vi "Linear Length 2 1478 1525 1828.vi"(0 "Input Image":T2, 1 "Calibration Image":T2, 5 "Ref ROI Parameters":T9={"Ref ROI After Transformation"={"Global Rectangle"=[], "Contours"=[]}, "Ref ROI Edge Options"={"Edge Polarity"=0, "Kernel Size"=3, "Width"=3, "Minimum Edge Strength"=10.0, "Interpolation Type"=enum."Zero Order", "Data Processing Method"=enum."Average"}, "Ref ROI Line Options"={"Number of Lines"=1, "Type"=enum."Best Edge Projection", "Min. Score"=0.0, "Max. Score"=1000.0, "Orientation"=0.0, "Angle Range"=5.0, "Angle Tolerance"=0.0, "Step Size"=5, "Min. SNR (db)"=0.0, "Min. Points (%)"=25.0, "Hough Iterations"=5}, "Ref ROI Search Direction"=0, "Ref ROI Overlay"=FALSE} {"Ref ROI Edge Options"."Edge Polarity" items=["All Edges", "Rising Edges", "Falling Edges"]; "Ref ROI Edge Options"."Minimum Edge Strength" format="%.2f"; "Ref ROI Edge Options"."Width" step=2; "Ref ROI Edge Options"."Kernel Size" step=2; "Ref ROI Line Options"."Min. Points (%)" min=0.0 max=100.0; "Ref ROI Line Options"."Min. SNR (db)" min=0.0; "Ref ROI Line Options"."Max. Score" min=0.0 max=1024.0; "Ref ROI Line Options"."Min. Score" min=0.0 max=1024.0 step=1.0}, 7 "ROI 1 Parameters":T6={"ROI 1 After Transformation"={"Global Rectangle"=[], "Contours"=[]}, "ROI 1 Edge Options"={"Edge Polarity"=0, "Kernel Size"=3, "Width"=3, "Minimum Edge Strength"=10.0, "Interpolation Type"=enum."Bilinear Fixed", "Data Processing Method"=enum."Average"}, "ROI 1 Scan Direction"=0, "ROI 1 Step Size"=0, "ROI 1 Process"=enum."Get First Edge", "ROI 1 Overlay"=FALSE, "ROI 1 Rake Line Overlay"=FALSE, "ROI 1 Edge/Point Overlay"=FALSE} {"ROI 1 Edge Options"."Edge Polarity" items=["All Edges", "Rising Edges", "Falling Edges"]; "ROI 1 Edge Options"."Minimum Edge Strength" format="%.2f"; "ROI 1 Edge Options"."Width" step=2; "ROI 1 Edge Options"."Kernel Size" step=2}, 9 "ROI 2 Parameters":T5={"ROI 2 After Transformation"={"Global Rectangle"=[], "Contours"=[]}, "ROI 2 Edge Options"={"Edge Polarity"=0, "Kernel Size"=3, "Width"=3, "Minimum Edge Strength"=10.0, "Interpolation Type"=enum."Bilinear Fixed", "Data Processing Method"=enum."Average"}, "ROI 2 Scan Direction"=0, "ROI 2 Step Size"=0, "ROI 2 Process"=enum."Get First Edge", "ROI 2 Overlay"=FALSE, "ROI 2 Rake Line Overlay"=FALSE, "ROI 2 Edge/Point Overlay"=FALSE} {"ROI 2 Edge Options"."Edge Polarity" items=["All Edges", "Rising Edges", "Falling Edges"]; "ROI 2 Edge Options"."Minimum Edge Strength" format="%.2f"; "ROI 2 Edge Options"."Width" step=2; "ROI 2 Edge Options"."Kernel Size" step=2}, 11 "error in (no error)":errorcluster) -> (4 "Refnum out":T2(plugin-control), 6 "output cluster":T10, 8 "Overlay Arrow Lines":T1, 15 "error out":errorcluster)   [LabVIEW 2019, in "Algorithm.lvclass"]
uses:
  FrameworkOverrides/Algorithm.lvclass
  <vilib>/vision/NI_Vision_Development_Module.lvlib
  <vilib>/vision/Measure.llb/Edge Polarity.ctl
  <vilib>/vision/Measure.llb/Edge Options.ctl
  <vilib>/vision/Measure.llb/Straight Edge Process.ctl
  <vilib>/vision/Measure.llb/Straight Edge Options.ctl
  <vilib>/vision/Image Controls.llb/IMAQ Image.ctl
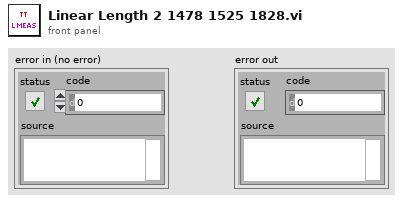
[diagram p1: front panel]
types:
  T1 = cluster{cluster{cluster{sgl, "Y":sgl}, "Point 2":cluster{"X":sgl, "Y":sgl}}, cluster{"Point 2":cluster{"X":sgl, "Y":sgl}, cluster{sgl, "Y":sgl}}}
  T2 = typedef "IMAQ Image.ctl" = refnum<image>
  T3 = typedef "Edge Options.ctl" = cluster{"Edge Polarity":T4, "Kernel Size":u32, "Width":u32, "Minimum Edge Strength":sgl, "Interpolation Type":enum32{"Zero Order", "Bilinear", "Quadratic", "Cubic", "Bilinear Fixed"}, "Data Processing Method":enum32{"Average", "Median"}}
  T4 = typedef "Edge Polarity.ctl" = u32
  T5 = cluster{"ROI 2 After Transformation":cluster{"Global Rectangle":i32[], "Contours":cluster{"ID":enum32{"External", "Internal"}, "Type":u32, "Coordinates":i32[]}[]}, "ROI 2 Edge Options":T3, "ROI 2 Scan Direction":u16, "ROI 2 Step Size":u32, "ROI 2 Process":enum16{"Get First Edge", "Get First + Last Edge", "Get All Edges", "Get Best Edge"}, "ROI 2 Overlay":bool, "ROI 2 Rake Line Overlay":bool, "ROI 2 Edge/Point Overlay":bool}
  T6 = cluster{"ROI 1 After Transformation":cluster{"Global Rectangle":i32[], "Contours":cluster{"ID":enum32{"External", "Internal"}, "Type":u32, "Coordinates":i32[]}[]}, "ROI 1 Edge Options":T3, "ROI 1 Scan Direction":u16, "ROI 1 Step Size":u32, "ROI 1 Process":enum16{"Get First Edge", "Get First + Last Edge", "Get All Edges", "Get Best Edge"}, "ROI 1 Overlay":bool, "ROI 1 Rake Line Overlay":bool, "ROI 1 Edge/Point Overlay":bool}
  T7 = typedef "Straight Edge Options.ctl" = cluster{"Number of Lines":i32, "Type":T8, "Min. Score":dbl, "Max. Score":dbl, "Orientation":dbl, "Angle Range":dbl, "Angle Tolerance":dbl, "Step Size":u32, "Min. SNR (db)":dbl, "Min. Points (%)":dbl, "Hough Iterations":i32}
  T8 = typedef "Straight Edge Process.ctl" = enum32{"First Edge Rake", "Best Edge Rake", "Hough Edge Rake", "First Edge Projection", "Best Edge Projection"}
  T9 = cluster{"Ref ROI After Transformation":cluster{"Global Rectangle":i32[], "Contours":cluster{"ID":enum32{"External", "Internal"}, "Type":u32, "Coordinates":i32[]}[]}, "Ref ROI Edge Options":T3, "Ref ROI Line Options":T7, "Ref ROI Search Direction":u32, "Ref ROI Overlay":bool}
  T10 = cluster{"L Meas":sgl, "output cluster":cluster{"Point 2":cluster{"X":sgl, "Y":sgl}, "Point 2":cluster{"X":sgl, "Y":sgl}}}
  T11 = cluster{"First Overlay Line ":cluster{"Start Point":cluster{"X":sgl, "Y":sgl}, "Start Point":cluster{"X":sgl, "Y":sgl}}, "Second Overlay Line ":cluster{"Start Point":cluster{"X":sgl, "Y":sgl}, "Start Point":cluster{"X":sgl, "Y":sgl}}}
  T12 = cluster{"Search Direction":u32, "Edge Options":T3, "Show Search Area":bool, "Show Search Lines":bool, "Show Edges Found":bool, "Show Result":bool, "Search Area Color":u32, "Search Lines Color":u32, "Edge Locations Color":u32, "Result Color":u32, "Overlay Group Name":string}
  T13 = cluster{"Global Rectangle":i32[], "Contours":cluster{"ID":enum32{"External", "Internal"}, "Type":u32, "Coordinates":i32[]}[]}
  T14 = enum16{"Get First Edge", "Get First + Last Edge", "Get All Edges", "Get Best Edge"}
  T15 = cluster{"Point1 (Pixels)":cluster{"X":sgl, "Y":sgl}, "Point2 (Pixels)":cluster{"X":sgl, "Y":sgl}, "Point1 (Real-World)":cluster{"X":sgl, "Y":sgl}, "Point2 (Real-World)":cluster{"X":sgl, "Y":sgl}, "Angle (Pixel)":dbl, "Angle (Real-World)":dbl, "Score":dbl, "Straightness":dbl, "Average SNR (db)":dbl, "Calibration Valid":bool}[]
  T16 = typedef "Edge New.ctl" = cluster{"Location (Pixel)":cluster{"X":sgl, "Y":sgl}, "Location (Real-World)":cluster{"X":sgl, "Y":sgl}, "Distance (Pixel)":dbl, "Distance (Real-World)":dbl, "Strength":dbl, "Noise":dbl, "Rising?":bool}
  T17 = typedef "Search Line.ctl" = cluster{"Start Point":cluster{"X":sgl, "Y":sgl}, "End Point":cluster{"X":sgl, "Y":sgl}, "Edge Info":T16[], "Edge Map":dbl[], "Calibration Valid":bool}
  T18 = cluster{"Point1 (Pixels)":cluster{"X":sgl, "Y":sgl}, "Point2 (Pixels)":cluster{"X":sgl, "Y":sgl}, "Point1 (Real-World)":cluster{"X":sgl, "Y":sgl}, "Point2 (Real-World)":cluster{"X":sgl, "Y":sgl}, "Angle (Pixel)":dbl, "Angle (Real-World)":dbl, "Score":dbl, "Straightness":dbl, "Average SNR (db)":dbl, "Calibration Valid":bool}
  T19 = cluster{"Point1 (Pixels)":cluster{"X":sgl, "Y":sgl}, "Point2 (Pixels)":cluster{"X":sgl, "Y":sgl}}
  T20 = cluster{"Point 1":cluster{"X":sgl, "Y":sgl}, "Point 2":cluster{"X":sgl, "Y":sgl}}
  T21 = cluster{"Point 2":cluster{"X":sgl, "Y":sgl}, "Point 2":cluster{"X":sgl, "Y":sgl}}
  T22 = cluster{cluster{sgl, "Y":sgl}, "Point 2":cluster{"X":sgl, "Y":sgl}}
  T23 = cluster{"Point 2":cluster{"X":sgl, "Y":sgl}, cluster{sgl, "Y":sgl}}
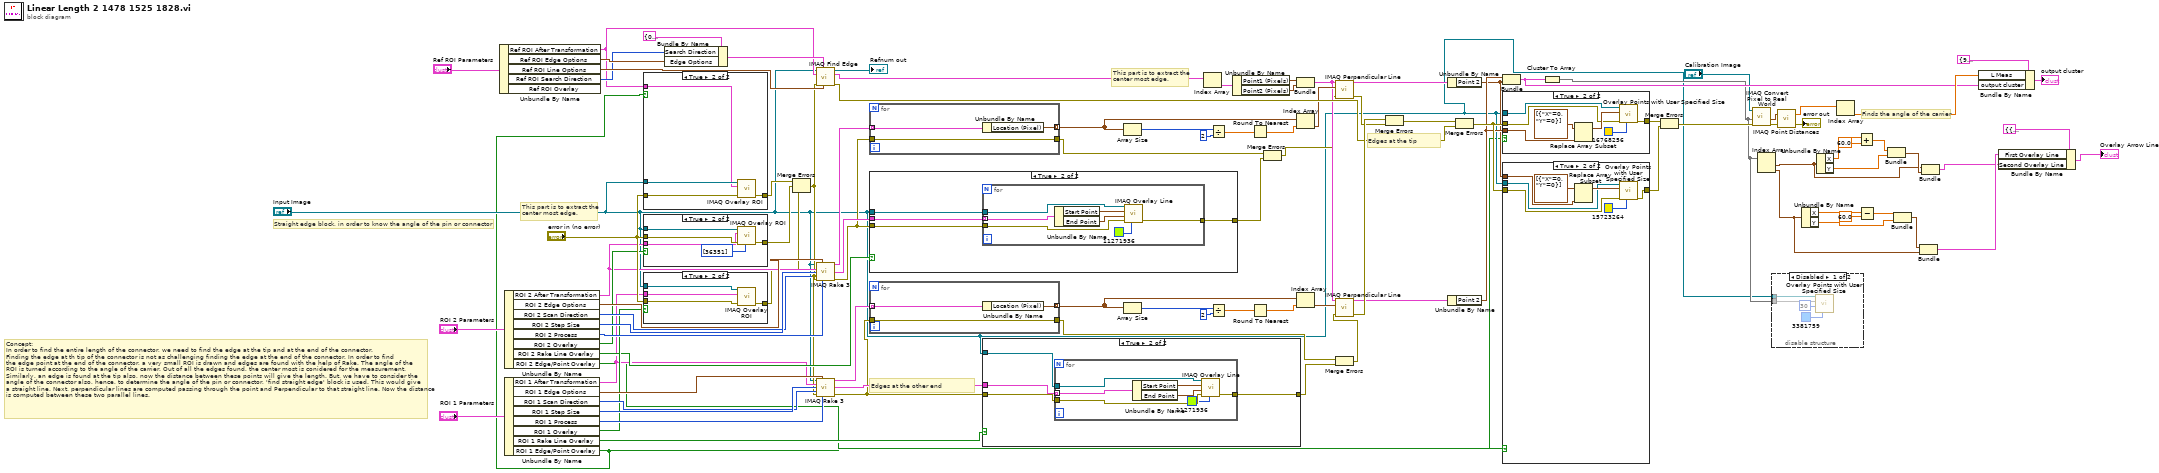
[diagram p0: block diagram]
diagram:
  # "Straight edge block, in order to know the angle of the pin or connector"
  # "This part is to extract the\ncenter most edge."
  # "This part is to extract the\ncenter most edge."
  # "Concept:\nIn order to find the entire length of the connector, we need to find the edge at the tip and at the end of the connector.\nFinding the edge at th tip of the connector is not as challenging finding the edge at the end of the connector. In order to find\nthe edge point at the end of the connector, a very small ROI is drawn and edges are found with the help of Rake. The angle of the \nROI is turned according to the angle of the carrier. Out of all the edges found, the center most is conidered for the measurement.\nSimilarly, an edge is found at the tip also, now the distance between these points will give the length. But, we have to consider the \nangle of the connector also, hence, to determine the angle of the pin or connector, 'find straight edge' block is used. This would give\na straight line. Next, perpendicular lines are computed passing through the point and Perpendicular to that straight line. Now the distance\nis computed between these two parallel lines."
  # "Finds the angle of the carrier"
  # "Edges at the other end"
  # "Edges at the tip"
  n1 = Unbundle By Name("Ref ROI Parameters") -> ("Ref ROI After Transformation"=w36:T13, "Ref ROI Edge Options"=w65:T3, "Ref ROI Line Options"=w66:T7, "Ref ROI Search Direction"=w64:u32)  [unwired: 1 out]
  n2 = Unbundle By Name("ROI 2 Parameters") -> ("ROI 2 After Transformation"=w47:T13, "ROI 2 Edge Options"=w63:T3, "ROI 2 Scan Direction"=w60:u16, "ROI 2 Step Size"=w61:u32, "ROI 2 Process"=w62:T14, "ROI 2 Overlay"=w48:bool, "ROI 2 Rake Line Overlay"=w44:bool, "ROI 2 Edge/Point Overlay"=w35:bool)
  n3 = Unbundle By Name("ROI 1 Parameters") -> ("ROI 1 After Transformation"=w37:T13, "ROI 1 Edge Options"=w59:T3, "ROI 1 Scan Direction"=w56:u16, "ROI 1 Step Size"=w57:u32, "ROI 1 Process"=w58:T14, "ROI 1 Overlay"=w50:bool, "ROI 1 Rake Line Overlay"=w43:bool, "ROI 1 Edge/Point Overlay"=w1:bool)
  n4 = case shown="True" w1 {
    tunnel: "error in (no error)" -> [w100 w104]
    tunnel: [w100 w103] -> w32
    tunnel: "Input Image" -> [_ w102]
    tunnel: w36 -> [_ w101]
    frame False {
    }
    frame True {
      n5 = call "IMAQ Overlay ROI"("error in (no error)"=w104, "ROI Descriptor"=w101, "Image"=w102) -> ("error out"=w103:errorcluster)  [unwired: 7 in, 1 out]
    }
  }
  n6 = case shown="True" w48 {
    tunnel: "error in (no error)" -> [w105 w110]
    tunnel: [w105 w109] -> w31
    tunnel: "Input Image" -> [_ w108]
    tunnel: w47 -> [_ w107]
    frame False {
    }
    frame True {
      n7 = call "IMAQ Overlay ROI"("Colors (Green)"=u32[] [36351], "error in (no error)"=w110, "ROI Descriptor"=w107, "Image"=w108) -> ("error out"=w109:errorcluster)  [unwired: 6 in, 1 out]
    }
  }
  n8 = case shown="True" w50 {
    tunnel: "error in (no error)" -> [w111 w115]
    tunnel: [w111 w114] -> w30
    tunnel: "Input Image" -> [_ w113]
    tunnel: w37 -> [_ w112]
    frame False {
    }
    frame True {
      n9 = call "IMAQ Overlay ROI"("error in (no error)"=w115, "ROI Descriptor"=w112, "Image"=w113) -> ("error out"=w114:errorcluster)  [unwired: 7 in, 1 out]
    }
  }
  n10 = Bundle By Name(cluster=T12 {"Search Direction"=0, "Edge Options"={"Edge Polarity"=0, "Kernel Size"=3, "Width"=3, "Minimum Edge Strength"=10.0, "Interpolation Type"=enum."Bilinear Fixed", "Data Processing Method"=enum."Average"}, "Show Search Area"=FALSE, "Show Search Lines"=FALSE, "Show Edges Found"=FALSE, "Show Result"=TRUE, "Search Area Color"=65280, "Search Lines Color"=255, "Edge Locations Color"=16776960, "Result Color"=65337, "Overlay Group Name"=""} ("Options"), "Search Direction"=w64, "Edge Options"=w65) -> (w70:T12)
  n11 = Merge Errors(w32, w31, w30) -> (w29:errorcluster)
  n12 = call "IMAQ Find Edge"("Line Fit Options"=w66, "Options"=w70, "error in (no error)"=w29, "ROI Descriptor"=w36, "Image"="Input Image") -> ("error out"=w95:errorcluster, "Straight Edges"=w90:T15, "Image Out"=→"Refnum out":T2)  [unwired: 3 in, 1 out]
  n13 = call "IMAQ Rake 3"("Image"="Input Image", "Edge Options"=w63, "ROI Descriptor"=w47, "Step Size"=w61, "Scan Direction"=w60, "error in (no error)"=w29, "Process"=w62) -> ("First Edges"=w81:T16[], "Search Lines"=w45:T17[], "error out"=w28:errorcluster)  [unwired: 5 in, 1 out]
  n14 = call "IMAQ Rake 3"("Image"="Input Image", "Edge Options"=w59, "ROI Descriptor"=w37, "Step Size"=w57, "Scan Direction"=w56, "error in (no error)"=w29, "Process"=w58) -> ("First Edges"=w20:T16[], "Search Lines"=w46:T17[], "error out"=w22:errorcluster)  [unwired: 5 in, 1 out]
  n15 = for {
    tunnel: w81 -> [w118] mode=indexing
    tunnel: [w117] -> w73 mode=indexing
    tunnel: w28 -> [w116]
    tunnel: [w116] -> w27
    n16 = Unbundle By Name(w118) -> ("Location (Pixel)"=w117:cluster{"X":sgl, "Y":sgl})
  }
  n17 = case shown="True" w44 {
    tunnel: [w119 w123] -> w26
    tunnel: w28 -> [w119 w122]
    tunnel: w45 -> [_ w121]
    tunnel: "Input Image" -> [_ w120]
    frame False {
    }
    frame True {
      n18 = for {
        tunnel: [w130] -> w123
        tunnel: w122 -> [w129]
        tunnel: w121 -> [w128] mode=indexing
        tunnel: w120 -> [w125]
        n19 = Unbundle By Name(w128) -> ("Start Point"=w127:cluster{"X":sgl, "Y":sgl}, "End Point"=w126:cluster{"X":sgl, "Y":sgl})
        n20 = call "IMAQ Overlay Line"("Color"=u32 11271936, "error in (no error)"=w129, "End Point"=w126, "Start Point"=w127, "Image"=w125) -> ("error out"=w130:errorcluster)  [unwired: 5 in, 1 out]
      }
    }
  }
  n21 = for {
    tunnel: w20 -> [w133] mode=indexing
    tunnel: [w132] -> w52 mode=indexing
    tunnel: w22 -> [w131]
    tunnel: [w131] -> w21
    n22 = Unbundle By Name(w133) -> ("Location (Pixel)"=w132:cluster{"X":sgl, "Y":sgl})
  }
  n23 = case shown="True" w43 {
    tunnel: [w134 w138] -> w24
    tunnel: w22 -> [w134 w137]
    tunnel: w46 -> [_ w136]
    tunnel: "Input Image" -> [_ w135]
    frame False {
    }
    frame True {
      n24 = for {
        tunnel: [w145] -> w138
        tunnel: w137 -> [w144]
        tunnel: w136 -> [w143] mode=indexing
        tunnel: w135 -> [w140]
        n25 = Unbundle By Name(w143) -> ("Start Point"=w142:cluster{"X":sgl, "Y":sgl}, "End Point"=w141:cluster{"X":sgl, "Y":sgl})
        n26 = call "IMAQ Overlay Line"("Color"=u32 11271936, "error in (no error)"=w144, "End Point"=w141, "Start Point"=w142, "Image"=w140) -> ("error out"=w145:errorcluster)  [unwired: 5 in, 1 out]
      }
    }
  }
  n27 = Array Size(array=w73) -> (size(s)=w89:i32)
  n28 = Array Size(array=w52) -> (size(s)=w82:i32)
  n29 = Index Array(array=w90) -> (element=w91:T18)  [unwired: 1 in]
  n30 = Divide(x=w89, y=2 ("index (row)")) -> (x/y=w87:dbl)
  n31 = Divide(x=w82, y=2 ("index (row)")) -> (x/y=w84:dbl)
  n32 = Unbundle By Name(w91) -> ("Point1 (Pixels)"=w75:cluster{"X":sgl, "Y":sgl}, "Point2 (Pixels)"=w74:cluster{"X":sgl, "Y":sgl})
  n33 = Round To Nearest(number=w87) -> (nearest integer value=w86:dbl)
  n34 = Round To Nearest(number=w84) -> (nearest integer value=w85:dbl)
  n35 = Merge Errors(w27, w26) -> (w25:errorcluster)
  n36 = Bundle("Point1 (Pixels)"=w75, "Point2 (Pixels)"=w74) -> (w92:T19)  [unwired: 1 in]
  n37 = Index Array(array=w73, index=w86) -> (element=w94:cluster{"X":sgl, "Y":sgl})
  n38 = Index Array(array=w52, index=w85) -> (element=w93:cluster{"X":sgl, "Y":sgl})
  n39 = call "IMAQ Perpendicular Line"("error in (no error)"=w25, "Point"=w94, "Line"=w92) -> ("error out"=w96:errorcluster, "Perpendicular Line"=w53:T20)  [unwired: 6 in, 1 out]
  n40 = Merge Errors(w21, w24) -> (w23:errorcluster)
  n41 = call "IMAQ Perpendicular Line"("error in (no error)"=w23, "Point"=w93, "Line"=w92) -> ("error out"=w97:errorcluster, "Perpendicular Line"=w54:T20)  [unwired: 6 in, 1 out]
  n42 = Merge Errors(w97, w96) -> (w98:errorcluster)
  n43 = Unbundle By Name(w53) -> ("Point 2"=w38:cluster{"X":sgl, "Y":sgl})
  n44 = Unbundle By Name(w54) -> ("Point 2"=w39:cluster{"X":sgl, "Y":sgl})
  n45 = Merge Errors(w98, w95) -> (w40:errorcluster)
  n46 = Bundle("Point 2"=w39, "Point 2"=w38) -> (w76:T21)  [unwired: 1 in]
  n47 = case shown="True" w1 {
    tunnel: [w146 w150] -> w42
    tunnel: w40 -> [w146 w151]
    tunnel: w39 -> [_ w149]
    tunnel: "Input Image" -> [_ w148]
    frame False {
    }
    frame True {
      n48 = Replace Array Subset(array=cluster{"X":i32, "Y":i32}[] [{"X"=0, "Y"=0}] ("Points"), new element=w149) -> (w152:cluster{"X":i32, "Y":i32}[])  [unwired: 1 in]
      n49 = call "Overlay Points with User Specified Size.vi"("Color"=u32 16768256, "error in"=w151, "Points"=w152, "Image In"=w148) -> ("error out"=w150:errorcluster)  [unwired: 6 in, 1 out]
    }
  }
  n50 = case shown="True" w35 {
    tunnel: [w154 w158] -> w41
    tunnel: w40 -> [w154 w159]
    tunnel: w38 -> [_ w157]
    tunnel: "Input Image" -> [_ w156]
    frame False {
    }
    frame True {
      n51 = Replace Array Subset(array=cluster{"X":i32, "Y":i32}[] [{"X"=0, "Y"=0}] ("Points"), new element=w157) -> (w160:cluster{"X":i32, "Y":i32}[])  [unwired: 1 in]
      n52 = call "Overlay Points with User Specified Size.vi"("Color"=u32 15723264, "error in"=w159, "Points"=w160, "Image In"=w156) -> ("error out"=w158:errorcluster)  [unwired: 6 in, 1 out]
    }
  }
  n53 = Cluster To Array(cluster=w76) -> (array=w15:cluster{"X":sgl, "Y":sgl}[])
  n54 = Merge Errors(w42, w41) -> (w34:errorcluster)
  n55 = call "IMAQ Convert Pixel to Real World"("error in (no error)"=w34, "Array of Pixel Coordinates"=w15, "Calibrated Image"="Calibration Image") -> ("error out"=w33:errorcluster, "Array of Real World Coordinates"=w72:cluster{"X":sgl, "Y":sgl}[])  [unwired: 3 in, 4 out]
  n56 = Index Array(array=w15) -> (element #1=w2:cluster{"X":sgl, "Y":sgl}, element #2=w10:cluster{"X":sgl, "Y":sgl})  [unwired: 2 in]
  n57 = disable-structure shown="Disabled" {
    disable-tunnel: w15 -> [w165 _]
    disable-tunnel: "Input Image" -> [w164 _]
    frame Disabled {
      n58 = call "Overlay Points with User Specified Size.vi"("Color"=u32 3381759, "Point Diameter (5)"=u32 30, "Points"=w165, "Image In"=w164) -> ()  [unwired: 6 in, 2 out]
    }
    frame Enabled {
    }
  }
  n59 = call "IMAQ Point Distances"("Points"=w72, "error in (no error)"=w33) -> ("Distances"=w99:sgl[], "error out"=→"error out":errorcluster)  [unwired: 3 in]
  n60 = Unbundle By Name(w10) -> ("X"=w18:sgl, "Y"=w16:sgl)
  n61 = Unbundle By Name(w2) -> ("X"=w6:sgl, "Y"=w19:sgl)
  n62 = Index Array(array=w99) -> (element=w78:sgl)  [unwired: 1 in]
  n63 = Add(x=w6, y=sgl 60.0) -> (x+y=w4:sgl)
  n64 = Subtract(x=w18, y=sgl 60.0) -> (x-y=w7:sgl)
  n65 = Bundle(w4, "Y"=w19) -> (w3:cluster{sgl, "Y":sgl})  [unwired: 1 in]
  n66 = Bundle(w7, "Y"=w16) -> (w11:cluster{sgl, "Y":sgl})  [unwired: 1 in]
  n67 = Bundle(w11, "Point 2"=w10) -> (w9:T22)  [unwired: 1 in]
  n68 = Bundle("Point 2"=w2, w3) -> (w8:T23)  [unwired: 1 in]
  n69 = Bundle By Name(cluster=T10 {"L Meas"=907.9092, "output cluster"={"Point 2"={"X"=0.0, "Y"=0.0}, "Point 2"={"X"=0.0, "Y"=0.0}}}, "L Meas"=w78, "output cluster"=w76) -> (→"output cluster":T10)
  n70 = Bundle By Name(cluster=T11 {"First Overlay Line "={"Start Point"={"X"=0.0, "Y"=0.0}, "Start Point"={"X"=0.0, "Y"=0.0}}, "Second Overlay Line "={"Start Point"={"X"=0.0, "Y"=0.0}, "Start Point"={"X"=0.0, "Y"=0.0}}} ("Overlay Arrows Lines"), "First Overlay Line"=w9, "Second Overlay Line"=w8) -> (→"Overlay Arrow Lines":T11)
